vi "switchboard_read_env.vi"(8 "error in":errorcluster, 11 "Handle":u32) -> (0 "error out":errorcluster, 2 "current time":timestamp, 3 "Handle out":u32, 4 "Probecard humidity":dbl, 5 "Matrix humidity":dbl, 6 "Probecard temperature":dbl, 7 "Matrix temperature":dbl)   [LabVIEW 2016]
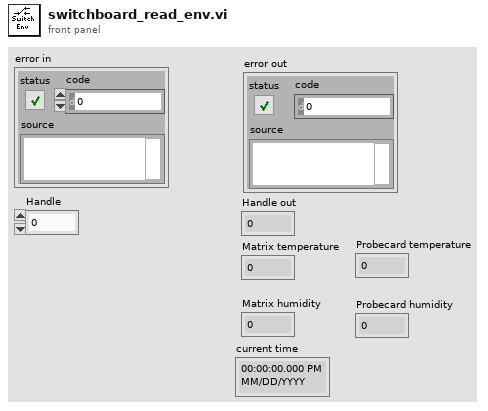
[diagram p1: front panel]
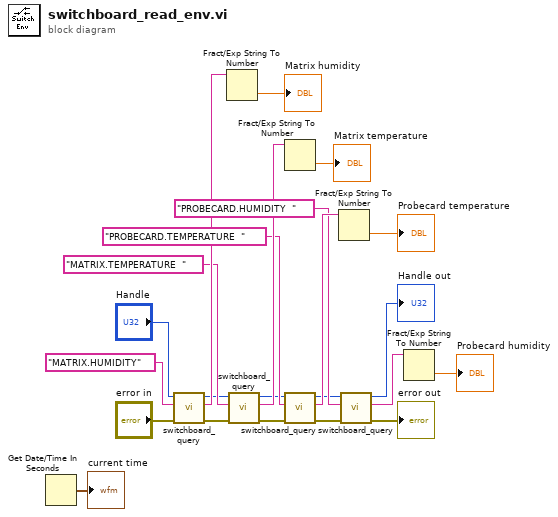
[diagram p0: block diagram]
diagram:
  n1 = Get Date/Time In Seconds() -> (seconds since 1Jan1904=→"current time":timestamp)
  n2 = call <instrlib>:"switchboard_query.vi"("error in"="error in", "Buffer"="MATRIX.HUMIDITY" ("string"), "Handle"="Handle") -> ("error out"=w13:errorcluster, "Read Buffer Out"=w20:string, "Handle"=w18:u32)  [unwired: 6 in]
  n3 = Fract/Exp String To Number(string=w20) -> (number=→"Matrix humidity":dbl)  [unwired: 3 in, 1 out]
  n4 = call <instrlib>:"switchboard_query.vi"("error in"=w13, "Buffer"="MATRIX.TEMPERATURE  " ("string"), "Handle"=w18) -> ("error out"=w4:errorcluster, "Read Buffer Out"=w17:string, "Handle"=w3:u32)  [unwired: 6 in]
  n5 = Fract/Exp String To Number(string=w17) -> (number=→"Matrix temperature":dbl)  [unwired: 3 in, 1 out]
  n6 = call <instrlib>:"switchboard_query.vi"("error in"=w4, "Buffer"="PROBECARD.TEMPERATURE  " ("string"), "Handle"=w3) -> ("error out"=w6:errorcluster, "Read Buffer Out"=w12:string, "Handle"=w5:u32)  [unwired: 6 in]
  n7 = Fract/Exp String To Number(string=w12) -> (number=→"Probecard temperature":dbl)  [unwired: 3 in, 1 out]
  n8 = call <instrlib>:"switchboard_query.vi"("error in"=w6, "Buffer"="PROBECARD.HUMIDITY  " ("string"), "Handle"=w5) -> ("error out"=→"error out":errorcluster, "Read Buffer Out"=w7:string, "Handle"=→"Handle out":u32)  [unwired: 6 in]
  n9 = Fract/Exp String To Number(string=w7) -> (number=→"Probecard humidity":dbl)  [unwired: 3 in, 1 out]
